vi "AccelerometerVoltageSampleLoop.vi"   [LabVIEW 2016]
uses:
  AccelerometerSample.ctl
  <vilib>/rvi/Emulation/niFpgaGetClockAttributes.vi
  <vilib>/rvi/Emulation/niFpgaSctlEmulationGetInTimedLoop.vi
  <vilib>/rvi/Emulation/niFpgaEmulationReportErrorSimple.vi
  <vilib>/rvi/Emulation/niFpgaEmulationIsFPGAContextNoSignature.vi
  <vilib>/rvi/errors/niFpgaSetErrorForExecOnDevCompSimple.vi
  <vilib>/rvi/eio/common/nirviEmuReportErrorAndStop.vi
  <vilib>/rvi/DataTransferAndStorage/Container/Common/niFpgaContainerGetUniqueNameForEmu.vi
  <vilib>/rvi/FIFO/Fifo_Resource/nirvififoEmulationSetSize.vi
  <vilib>/rvi/FIFO/Fifo_Resource/nirviFifoEmulationQueueMgr.vi
  <instcachedir>/0/nirviFifoEmulationQueueMgr_E5CAEC123FF24DC58D834DCA3CDAA9B5.lvgen/nirviFifoEmulationQueueMgr_E5CAEC123FF24DC58D834DCA3CDAA9B5_004.vi
  <vilib>/Utility/error.llb/Clear Errors.vi
  <vilib>/rvi/FIFO/Fifo_Resource/nirvififoEmulationCreateLock.vi
  <vilib>/rvi/Emulation/niFpgaProcessEmulError.vi
  <vilib>/rvi/FIFO/Fifo_Resource/nirvififoEmulationObtainLock.vi
  <vilib>/rvi/FIFO/Fifo_Resource/nirvififoEmulationReleaseLock.vi
  <vilib>/rvi/occurrence/nirviWaitOnOccurrenceBase.vi
  <vilib>/rvi/errors/nirviReportUnexpectedCaseInternalError.vi
  <vilib>/rvi/errors/nirviReportUnexpectedCaseInternalError (U32).vi
  <vilib>/rvi/eio/common/nirviEmuTemplateMethod_errors.vi
  <vilib>/rvi/Memory/Memory_Emulation/niFpgaMemoryEmulationCacheClearOnFirstRun.vi
  <vilib>/rvi/Memory/Memory_Emulation/nirvimemoryEmulationManagerCache_MakeExclusive.vi
  <vilib>/rvi/Memory/Memory_Emulation/niFpgaMemoryEmulationValidateCache.vi
  <vilib>/rvi/Memory/Memory_Emulation/nirvimemoryEmulationManagerCache_InsertValue.vi
  <vilib>/rvi/Memory/Memory_Emulation/nirvimemoryEmulationManagerCache_ReleaseExclusive.vi
  <vilib>/rvi/Memory/Memory_Emulation/nirvimemoryEmulationManagerCache_GetValue.vi
  <vilib>/rvi/Memory/Memory_Emulation/nirvimemoryEmulationManagerCache_SetValue.vi
  <instcachedir>/0/nirviFifoEmulationQueueMgr_E5CAEC123FF24DC58D834DCA3CDAA9B5.lvgen/nirviFifoEmulationQueueMgr_E5CAEC123FF24DC58D834DCA3CDAA9B5_044.vi
  <vilib>/rvi/FIFO/Fifo_Resource/nirvififoEmulationDetermineInputValidOut.vi
  <vilib>/rvi/Emulation/niFpgaCriticalErrorInLSC.vi
  <vilib>/rvi/DataTransferAndStorage/Container/XNode/niFpgaContainer.xnode
  <vilib>/rvi/FIFO/Fifo_Resource/nirvififoEmulationRead.vi
  <vilib>/eio/EIONode/EIONode.xnode
  <vilib>/rvi/DataTransferAndStorage/Register/Emulation/niFpgaRegisterEmulation.vi
  <vilib>/rvi/FIFO/Fifo_Resource/nirvififoEmulationWrite.vi
types:
  T1 = typedef "AccelerometerSample.ctl" = cluster{"Sample":u64, "Timestamp":u64, "Raw1":sgl, "Raw2":sgl, "Raw3":sgl, "Raw4":sgl, "Raw5":sgl, "Raw6":sgl, "Raw7":sgl, "Raw8":sgl}
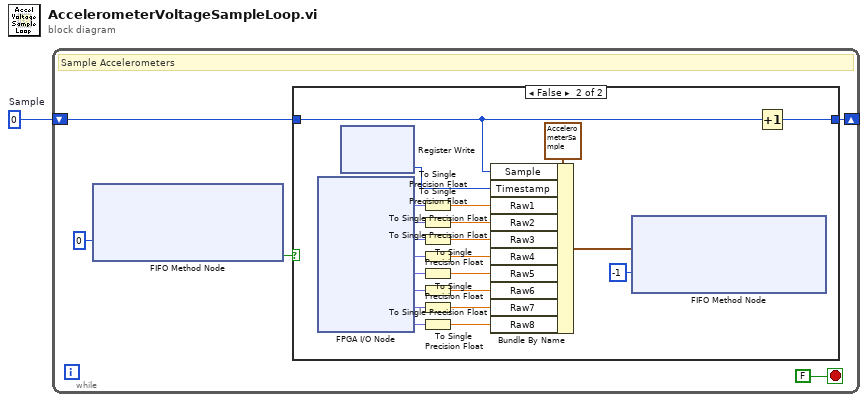
[diagram p0: block diagram]
diagram:
  w1 = u64 0  # Sample
  n1 = while {
    shift-right: [w2] -> _
    shift-left: w1 -> [w3]
    stop <- FALSE stop-if-true
    # "Sample Accelerometers"
    n2 = xnode ("FIFO Method Node")("Timeout"=0) -> ("Timed Out?"=w5:bool)  [unwired: 1 in, 2 out]
    n3 = case shown="False" w5 {
      tunnel: w3 -> [w7 w10]
      tunnel: [w7 w9] -> w2
      frame True {
      }
      frame False {
        n4 = xnode "FPGA I/O Node"() -> ("Mod1/AI0"=w29:fxp<+/-,24,5>, "Mod1/AI1"=w28:fxp<+/-,24,5>, "Mod1/AI2"=w27:fxp<+/-,24,5>, "Mod1/AI3"=w26:fxp<+/-,24,5>, "Mod2/AI0"=w25:fxp<+/-,24,5>, "Mod2/AI1"=w24:fxp<+/-,24,5>, "Mod2/AI2"=w23:fxp<+/-,24,5>, "Mod2/AI3"=w22:fxp<+/-,24,5>)  [unwired: 8 in, 8 out]
        n5 = xnode "Register Write"() -> ("Data"=w8:u64)  [unwired: 1 in, 1 out]
        n6 = To Single Precision Float(number=w29) -> (single precision float=w21:sgl)
        n7 = To Single Precision Float(number=w28) -> (single precision float=w20:sgl)
        n8 = To Single Precision Float(number=w27) -> (single precision float=w19:sgl)
        n9 = To Single Precision Float(number=w26) -> (single precision float=w18:sgl)
        n10 = To Single Precision Float(number=w25) -> (single precision float=w17:sgl)
        n11 = To Single Precision Float(number=w24) -> (single precision float=w16:sgl)
        n12 = To Single Precision Float(number=w23) -> (single precision float=w15:sgl)
        n13 = To Single Precision Float(number=w22) -> (single precision float=w14:sgl)
        n14 = Bundle By Name(cluster=T1 {"Sample"=0, "Timestamp"=0, "Raw1"=0.0, "Raw2"=0.0, "Raw3"=0.0, "Raw4"=0.0, "Raw5"=0.0, "Raw6"=0.0, "Raw7"=0.0, "Raw8"=0.0} ("AccelerometerSample"), "Sample"=w10, "Timestamp"=w8, "Raw1"=w21, "Raw2"=w20, "Raw3"=w19, "Raw4"=w18, "Raw5"=w17, "Raw6"=w16, "Raw7"=w15, "Raw8"=w14) -> (w13:T1)
        n15 = xnode ("FIFO Method Node")("Element"=w13, "Timeout"=-1) -> ()  [unwired: 1 in, 2 out]
        n16 = Increment(x=w10) -> (x+1=w9:u64)
      }
    }
  }
